vi "Receiver UI.vi"() -> ()   [LabVIEW 2023, in "Receiver.lvclass"]
uses:
  Receiver.lvclass
  Controls/Operation.ctl
  Controls/State Cluster.ctl
  Controls/User Event Operation.ctl
  Controls/Receiver Data Cluster.ctl
  Downloads/Sample PC Template/Sample PC Template/Typedefs/Data.ctl
  Receiver.lvclass/Receiver.ctl
  Downloads/Sample PC Template/Sample PC Template/Sample PC Template.lvlib
panel:
  out "Receiver UI Trigered":bool
  out "Data":variant
  out "error out":errorcluster
  in  "error in (no error)":errorcluster
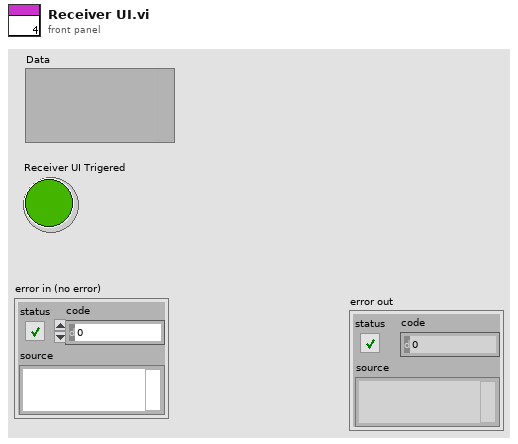
[diagram p1: front panel]
types:
  T1 = typedef "User Event Operation.ctl" = enum16{"Obtain", "Generate", "Release"}
  T2 = typedef "Receiver Data Cluster.ctl" = cluster{"Data":variant, "Receiver UI Triggered":bool}
  T3 = typedef "State Cluster.ctl" = cluster{"State":string, "Data":variant}
  T4 = typedef "Operation.ctl" = enum16{"Create", "Enqueue", "Enqueue N", "Enstack", "Dequeue", "Flush", "Release"}
  T5 = typedef "Sample PC Template.lvlib/Data.ctl" = cluster{"State":string, "Data":variant}
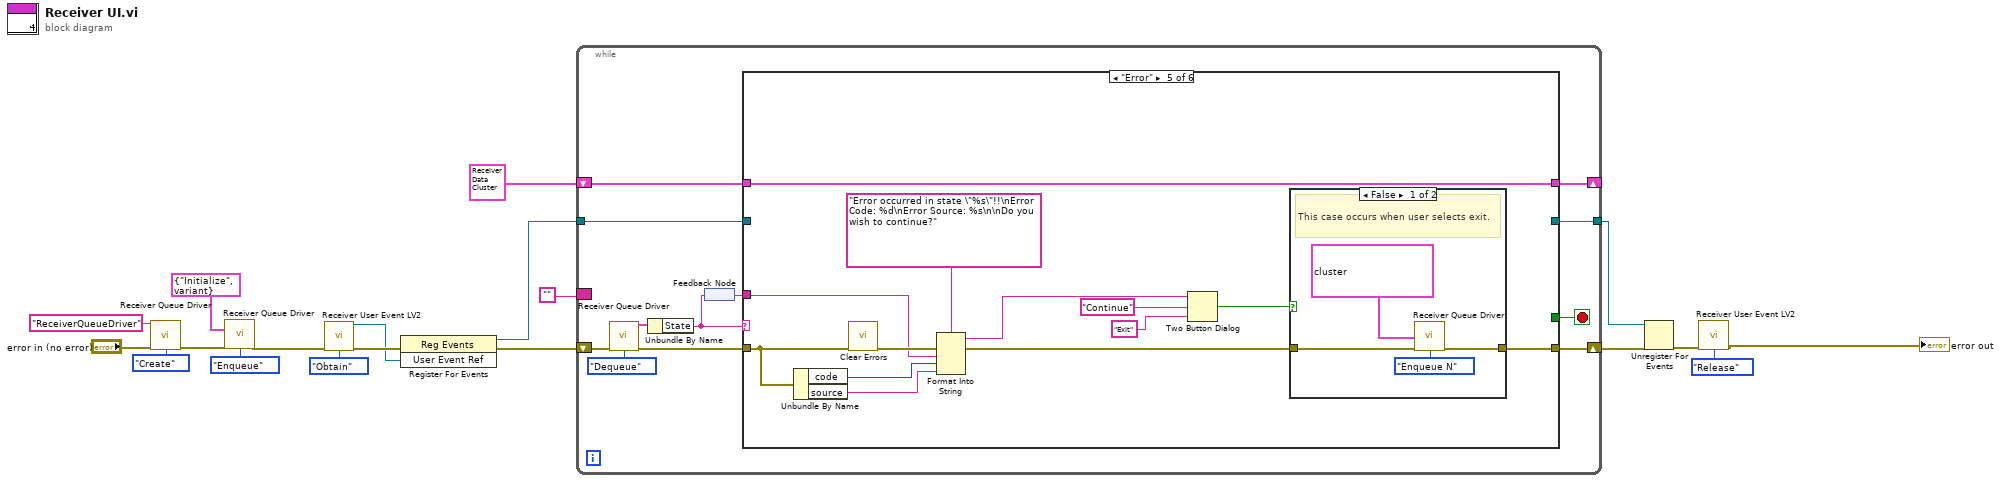
[diagram p0: block diagram]
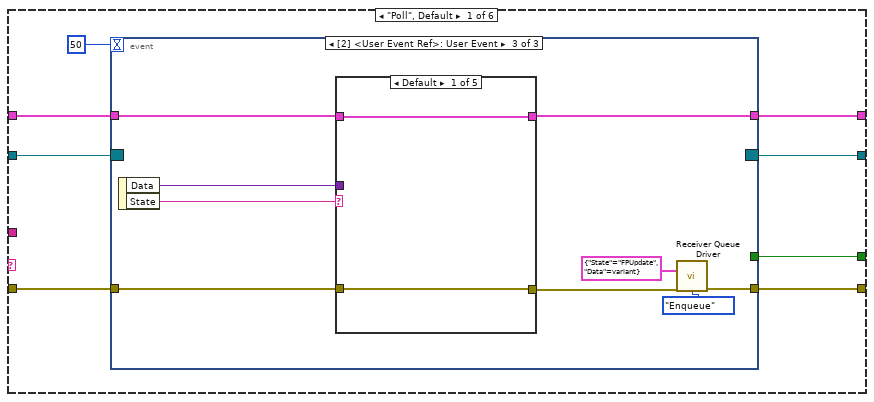
[diagram p2: hidden frame]
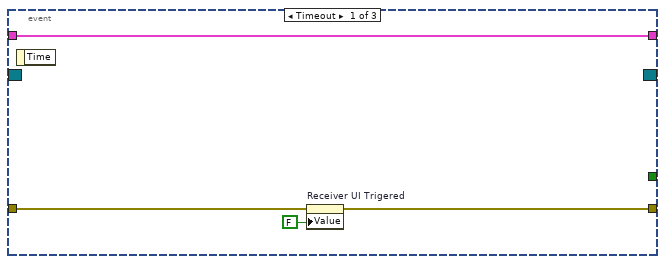
[diagram p3: hidden frame]
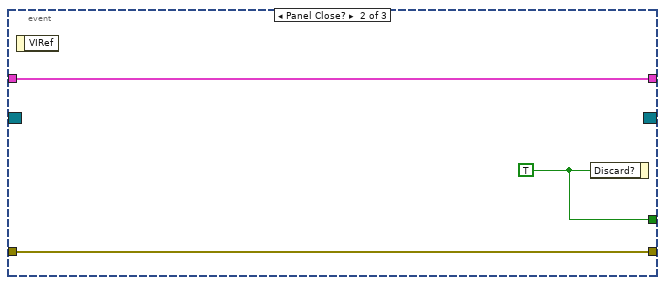
[diagram p4: hidden frame]
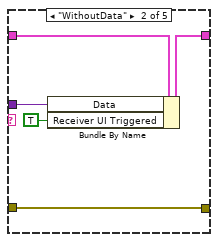
[diagram p5: hidden frame]
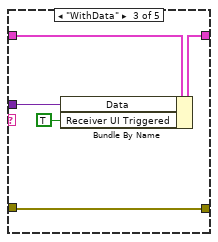
[diagram p6: hidden frame]
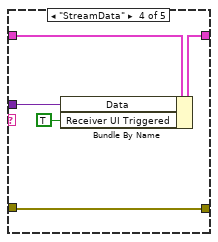
[diagram p7: hidden frame]
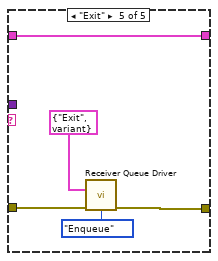
[diagram p8: hidden frame]
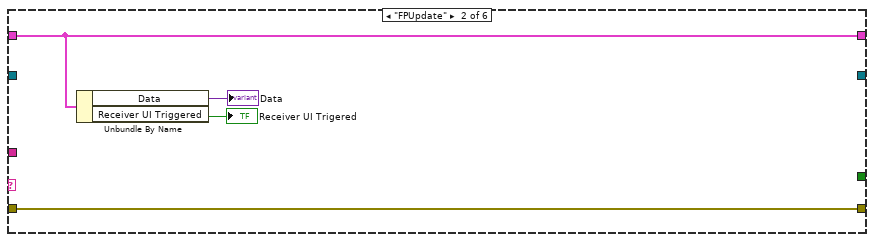
[diagram p9: hidden frame]
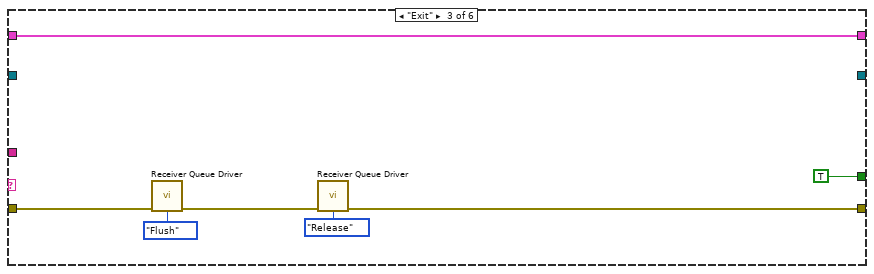
[diagram p10: hidden frame]
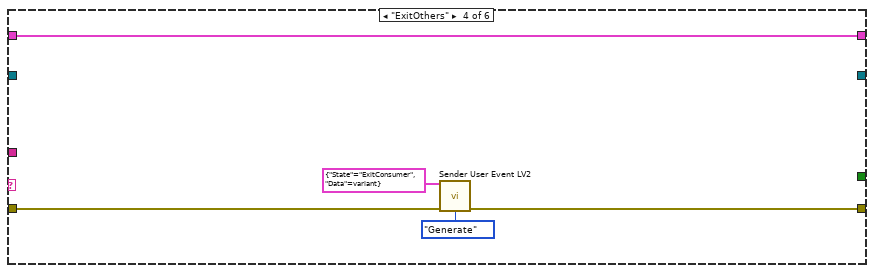
[diagram p11: hidden frame]
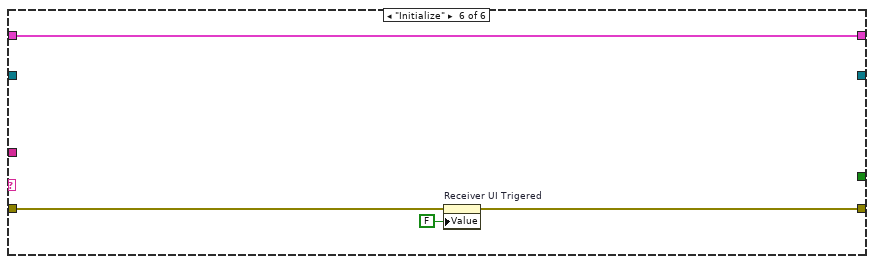
[diagram p13: hidden frame]
diagram:
  n1 = call "Receiver Queue Driver.vi"("Queue Name"="ReceiverQueueDriver", "error in (no error)"="error in (no error)", "Operations"=Operation."Create") -> ("error out"=w18:errorcluster)  [unwired: 11 in, 1 out]
  n2 = call "Receiver Queue Driver.vi"("State"=T3 {"State"="Initialize", "Data"=variant}, "error in (no error)"=w18, "Operations"=Operation."Enqueue") -> ("error out"=w12:errorcluster)  [unwired: 11 in, 1 out]
  n3 = call "Receiver User Event LV2.vi"("Error In"=w12, "Operation"=User_Event_Operation."Obtain") -> ("User Event Ref"=w8:refnum<user-event>, "Error Out"=w11:errorcluster)  [unwired: 12 in]
  n4 = register-events(error in=w11, w8) -> (reference out=w7:refnum<event-registration>, error out=w9:errorcluster)  [unwired: 1 in]
  n5 = while {
    border: "" -> [_]
    shift-right: [w25] -> w5
    shift-left: w9 -> [w30]
    tunnel: w7 -> [w23]
    shift-right: [w21] -> _
    shift-left: T2 {"Data"=variant, "Receiver UI Triggered"=FALSE} -> [w22]
    tunnel: [w20] -> w4
    stop <- w24 stop-if-true
    n6 = call "Receiver Queue Driver.vi"("error in (no error)"=w30, "Operations"=Operation."Dequeue") -> ("Dequeued Element"=w29:T3, "error out"=w28:errorcluster)  [unwired: 12 in]
    n7 = Unbundle By Name(w29) -> ("State"=w27:string)
    n8 = feedback-in #1(w27) -> ()
    n9 = feedback #1() -> (w26:string)
    n10 = case shown="\"Error\"" w27 {
      tunnel: w28 -> [w39 w81 w88 w93 w98 w114]
      tunnel: w26 -> [_ _ _ _ w95 _]
      tunnel: [w37 w81 w85 w92 w99 w112] -> w25
      tunnel: [w36 _ TRUE ("Discard?") _ _ _] -> w24
      tunnel: w23 -> [w35 _ _ _ _ _]
      tunnel: w22 -> [w34 w79 w82 w89 w94 w115]
      tunnel: [w33 w79 w82 w89 w94 w115] -> w21
      tunnel: [w32 _ _ _ _ _] -> w20
      frame "Poll", Default {
        n11 = event shown="[2] <User Event Ref>: User Event" {
          selector: w35 -> [_ _ _]
          dyn-events: [_ _ _] -> w32
          timeout: 50 -> [_ _ _]
          tunnel: w39 -> [w42 w46 w49]
          tunnel: [w41 w46 w52] -> w37
          tunnel: [_ w45 _] -> w36
          tunnel: w34 -> [w43 w44 w55]
          tunnel: [w43 w44 w53] -> w33
          event Timeout {
            n12 = event-data() -> ()  [unwired: 1 in, 1 out]
            n13 = property on="Receiver UI Trigered" class="Bool (strict)"(error in=w42, "Value"=FALSE ("Receiver UI Trigered")) -> (error out=w41:errorcluster)  [unwired: 1 in, 1 out]
          }
          event Panel Close? {
            w45 = TRUE ("Discard?")
            n14 = event-data() -> ()  [unwired: 1 in, 1 out]
            n15 = event-data("Discard?"=w45) -> ()  [unwired: 1 in, 1 out]
          }
          event User Event {
            n16 = event-data() -> ("Data"=w54:variant, "State"=w50:string)  [unwired: 1 in]
            n17 = case shown="Default" w50 {
              tunnel: w55 -> [w56 w62 w67 w72 w77]
              tunnel: w54 -> [_ w60 w66 w71 _]
              tunnel: [w56 w61 w65 w70 w77] -> w53
              tunnel: w49 -> [w57 w59 w63 w68 w76]
              tunnel: [w57 w59 w63 w68 w75] -> w48
              frame Default {
              }
              frame "WithoutData" {
                n18 = Bundle By Name(cluster=w62, "Data"=w60, "Receiver UI Triggered"=TRUE) -> (w61:T2)
              }
              frame "WithData" {
                n19 = Bundle By Name(cluster=w67, "Data"=w66, "Receiver UI Triggered"=TRUE) -> (w65:T2)
              }
              frame "StreamData" {
                n20 = Bundle By Name(cluster=w72, "Data"=w71, "Receiver UI Triggered"=TRUE) -> (w70:T2)
              }
              frame "Exit" {
                n21 = call "Receiver Queue Driver.vi"("State"=T3 {"State"="Exit", "Data"=variant}, "error in (no error)"=w76, "Operations"=Operation."Enqueue") -> ("error out"=w75:errorcluster)  [unwired: 11 in, 1 out]
              }
            }
            n22 = call "Receiver Queue Driver.vi"("State"=T3 {"State"="FPUpdate", "Data"=variant}, "error in (no error)"=w48, "Operations"=Operation."Enqueue") -> ("error out"=w52:errorcluster)  [unwired: 11 in, 1 out]
          }
        }
      }
      frame "FPUpdate" {
        n23 = Unbundle By Name(w79) -> ("Data"=→"Data":variant, "Receiver UI Triggered"=→"Receiver UI Trigered":bool)
      }
      frame "Exit" {
        n24 = call "Receiver Queue Driver.vi"("error in (no error)"=w88, "Operations"=Operation."Flush") -> ("error out"=w86:errorcluster)  [unwired: 12 in, 1 out]
        n25 = call "Receiver Queue Driver.vi"("error in (no error)"=w86, "Operations"=Operation."Release") -> ("error out"=w85:errorcluster)  [unwired: 12 in, 1 out]
      }
      frame "ExitOthers" {
        n26 = call "Sender User Event LV2.vi"("Data"=T5 {"State"="ExitConsumer", "Data"=variant}, "Error In"=w93, "Operation"=User_Event_Operation."Generate") -> ("Error Out"=w92:errorcluster)  [unwired: 11 in, 1 out]
      }
      frame "Error" {
        n27 = Unbundle By Name(w98) -> ("code"=w96:i32, "source"=w97:string)
        n28 = call <vilib>:"Clear Errors.vi"("error in (no error)"=w98) -> ("error out"=w106:errorcluster)  [unwired: 5 in, 1 out]
        n29 = Format Into String(format string="Error occurred in state \"%s\"!!\nError Code: %d\nError Source: %s\n\nDo you wish to continue?", error in=w106, w95, w96, w97) -> (resulting string=w104:string, error out=w101:errorcluster)  [unwired: 1 in]
        n30 = Two Button Dialog(message=w104, 1:"Exit" ("F button name (\"Cancel\")"), 2:"Continue" ("T button name (\"OK\")")) -> (T button?=w100:bool)
        n31 = case shown="False" w100 {
          tunnel: w101 -> [w110 w111]
          tunnel: [w109 w111] -> w99
          frame False {
            # "This case occurs when user selects exit."
            n32 = call "Receiver Queue Driver.vi"("State []"=T3[] [{"State"="ExitOthers", "Data"=variant}, {"State"="Exit", "Data"=variant}], "error in (no error)"=w110, "Operations"=Operation."Enqueue N") -> ("error out"=w109:errorcluster)  [unwired: 11 in, 1 out]
          }
          frame True {
            # "This case occurs when user selects to continue."
          }
        }
      }
      frame "Initialize" {
        n33 = property on="Receiver UI Trigered" class="Bool (strict)"(error in=w114, "Value"=FALSE ("Receiver UI Trigered")) -> (error out=w112:errorcluster)  [unwired: 1 in, 1 out]
      }
    }
  }
  n34 = Unregister For Events(event registration refnum=w4, error in=w5) -> (error out=w3:errorcluster)
  n35 = call "Receiver User Event LV2.vi"("Error In"=w3, "Operation"=User_Event_Operation."Release") -> ("Error Out"=→"error out":errorcluster)  [unwired: 12 in, 1 out]
